vi "Connection Response Offsets DAO.vi"(0 "Actions":T4, 3 "Config Ref Number":T3, 5 "LBCB Number":T1, 7 "Offsets In":T2, 11 "error in (no error)":errorcluster) -> (8 "Offsets Out":T2, 14 "Config Ref Number out":T3, 15 "error out":errorcluster)   [LabVIEW 2009]
uses:
  Metadata/Persistant DAO Actions.ctl
  Metadata/Cartesian Point.ctl
  <vilib>/Utility/config.llb/Config Data RefNum.ctl
  Metadata/LBCB Number.ctl
  <vilib>/Utility/config.llb/NI_LVConfig.lvlib
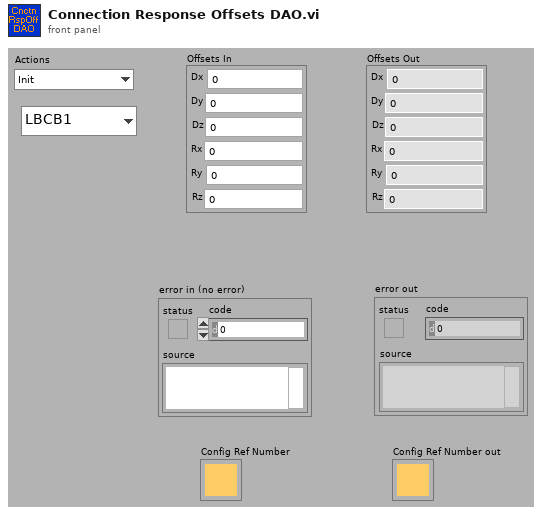
[diagram p1: front panel]
types:
  T1 = typedef "LBCB Number.ctl" = enum16{"LBCB1", "LBCB2"}
  T2 = typedef "Cartesian Point.ctl" = cluster{"Dx":dbl, "Dy":dbl, "Dz":dbl, "Rx":dbl, "Ry":dbl, "Rz":dbl}
  T3 = typedef "NI_LVConfig.lvlib/Config Data RefNum.ctl" = refnum<k1>
  T4 = typedef "Persistant DAO Actions.ctl" = enum16{"Init", "Get", "Set", "Load", "Save"}
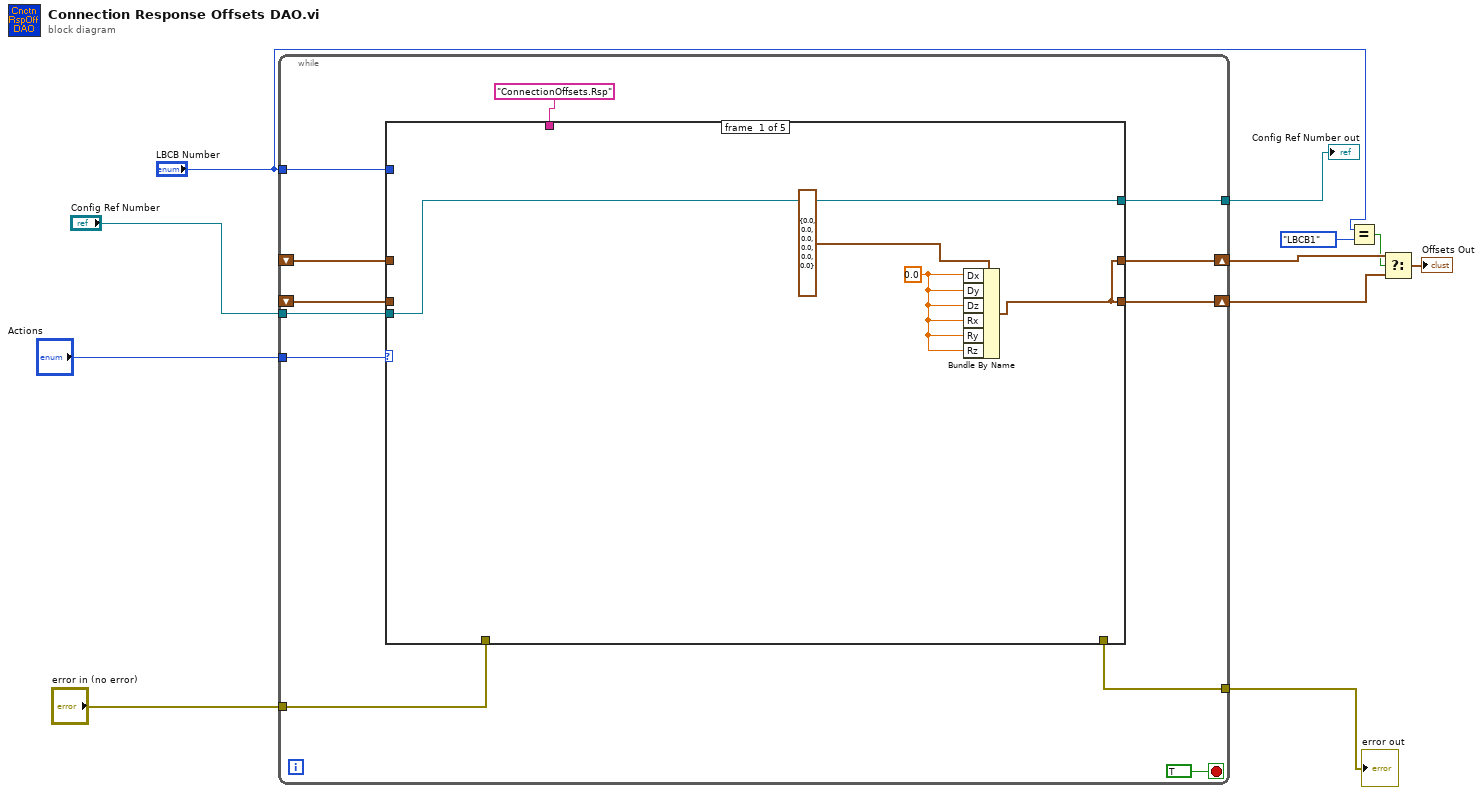
[diagram p0: block diagram]
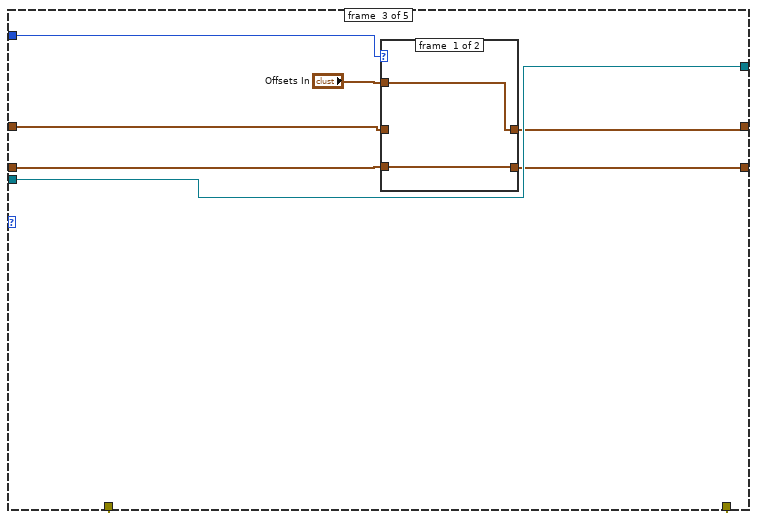
[diagram p3: hidden frame]
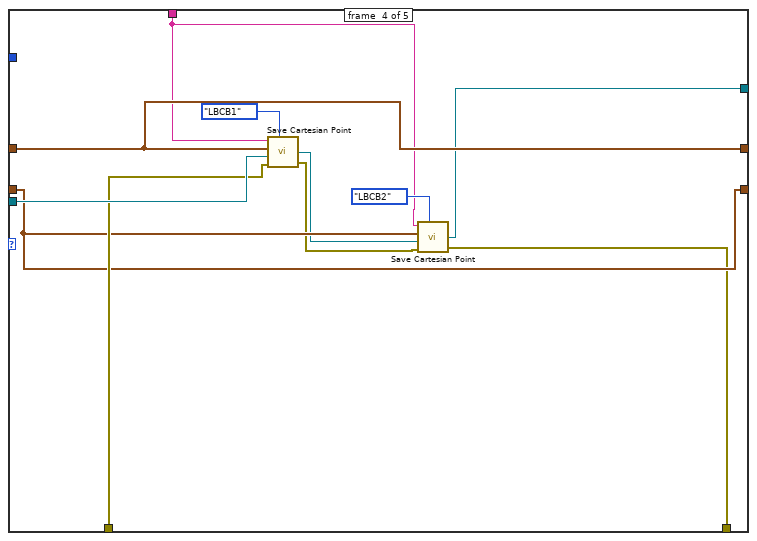
[diagram p5: hidden frame]
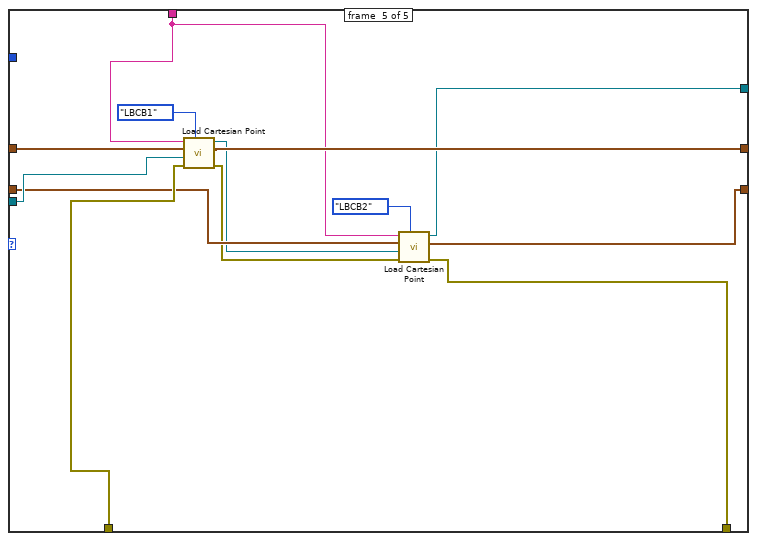
[diagram p6: hidden frame]
diagram:
  n1 = while {
    tunnel: "Actions" -> [w22]
    tunnel: "Config Ref Number" -> [w21]
    tunnel: "error in (no error)" -> [w19]
    tunnel: [w18] -> w8
    tunnel: [w17] -> w7
    shift-right: [w16] -> w5
    shift-left: _ -> [w15]
    tunnel: "LBCB Number" -> [w14]
    shift-right: [w13] -> w4
    shift-left: _ -> [w12]
    stop <- TRUE stop-if-true
    n2 = case shown="\"Init\"" w22 {
      tunnel: "ConnectionOffsets.Rsp" ("section") -> [_ _ _ w50 w62]
      tunnel: w21 -> [w27 w31 w39 w55 w68]
      tunnel: w19 -> [w28 w32 w40 w54 w67]
      tunnel: [w27 w31 w39 w47 w59] -> w18
      tunnel: [w28 w32 w40 w45 w57] -> w17
      tunnel: [w25 w30 w33 w53 w65] -> w16
      tunnel: w15 -> [_ w30 w36 w53 w66]
      tunnel: w14 -> [_ _ w38 _ _]
      tunnel: [w25 w29 w34 w49 w56] -> w13
      tunnel: w12 -> [_ w29 w35 w49 w61]
      frame #0 {
        w24 = 0.0 ("X")
        n3 = Bundle By Name(cluster=T2 {"Dx"=0.0, "Dy"=0.0, "Dz"=0.0, "Rx"=0.0, "Ry"=0.0, "Rz"=0.0} ("Max Increment Out"), "Dx"=w24, "Dy"=w24, "Dz"=w24, "Rx"=w24, "Ry"=w24, "Rz"=w24) -> (w25:T2)
      }
      frame #1 {
      }
      frame #2 {
        n4 = case shown="\"LBCB1\"" w38 {
          tunnel: "Offsets In" -> [w42 w44]
          tunnel: w36 -> [_ w43]
          tunnel: w35 -> [w41 _]
          tunnel: [w41 w44] -> w34
          tunnel: [w42 w43] -> w33
          frame #0 {
          }
          frame #1 {
          }
        }
      }
      frame #3 {
        n5 = call "Save Cartesian Point.vi"("section"=w50, "Input Cluster"=w53, "refnum"=w55, "error in (no error)"=w54, "LBCB Number"=LBCB_Number."LBCB1") -> ("refnum out"=w48:T3, "error out"=w46:errorcluster)  [unwired: 1 out]
        n6 = call "Save Cartesian Point.vi"("section"=w50, "Input Cluster"=w49, "refnum"=w48, "error in (no error)"=w46, "LBCB Number"=LBCB_Number."LBCB2") -> ("refnum out"=w47:T3, "error out"=w45:errorcluster)  [unwired: 1 out]
      }
      frame #4 {
        n7 = call "Load Cartesian Point.vi"("LBCB Number"=LBCB_Number."LBCB1", "error in (no error)"=w67, "refnum"=w68, "Input Cluster"=w66, "section"=w62) -> ("error out"=w58:errorcluster, "output cluster"=w65:T2, "refnum out"=w60:T3)  [unwired: 1 out]
        n8 = call "Load Cartesian Point.vi"("LBCB Number"=LBCB_Number."LBCB2", "error in (no error)"=w58, "refnum"=w60, "Input Cluster"=w61, "section"=w62) -> ("error out"=w57:errorcluster, "output cluster"=w56:T2, "refnum out"=w59:T3)  [unwired: 1 out]
      }
    }
  }
  "error out" <- w7
  "Config Ref Number out" <- w8
  n9 = Equal?(x="LBCB Number", y=LBCB_Number."LBCB1") -> (x = y?=w3:bool)
  n10 = Select(t=w5, s=w3, f=w4) -> (s? t:f=→"Offsets Out":T2)
